vi "createPartsTracking.vi"(0 "reference in":refnum<class "PartsTracking Controller.lvclass">, 5 "error in (no error)":errorcluster) -> (14 "reference out":refnum<class "PartsTracking Controller.lvclass">, 19 "error out":errorcluster)   [LabVIEW 2016, in "PartsTracking Controller.lvclass"]
uses:
  PartsTracking Controller.lvclass
  APP/partsTracking_class/partsTracking.lvclass
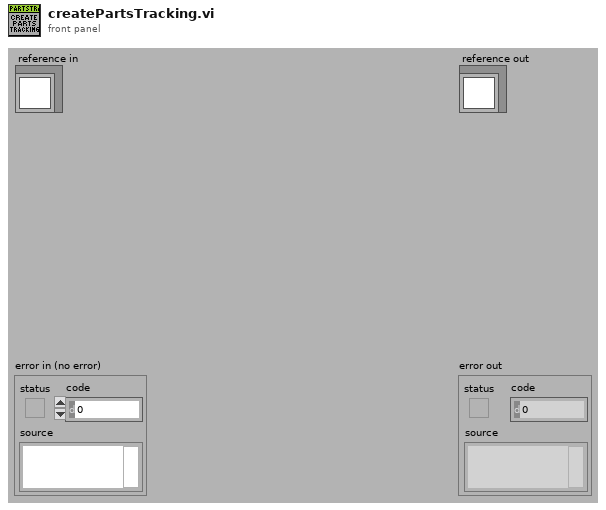
[diagram p1: front panel]
types:
  T1 = typedef "PartsTracking Controller.lvclass/ObjectAttributesRef.ctl" = refnum<data-value>
  T2 = typedef "PartsTracking Controller.lvclass/ObjectAttributes.ctl" = cluster{"MyAttribute":dbl, "file_controller_ref":refnum<class "File Controller.lvclass">, "data":string[][], "partsTracking_ref":refnum<class "partsTracking.lvclass">, "project_panels_ref":refnum<class "Project Panels.lvclass">}
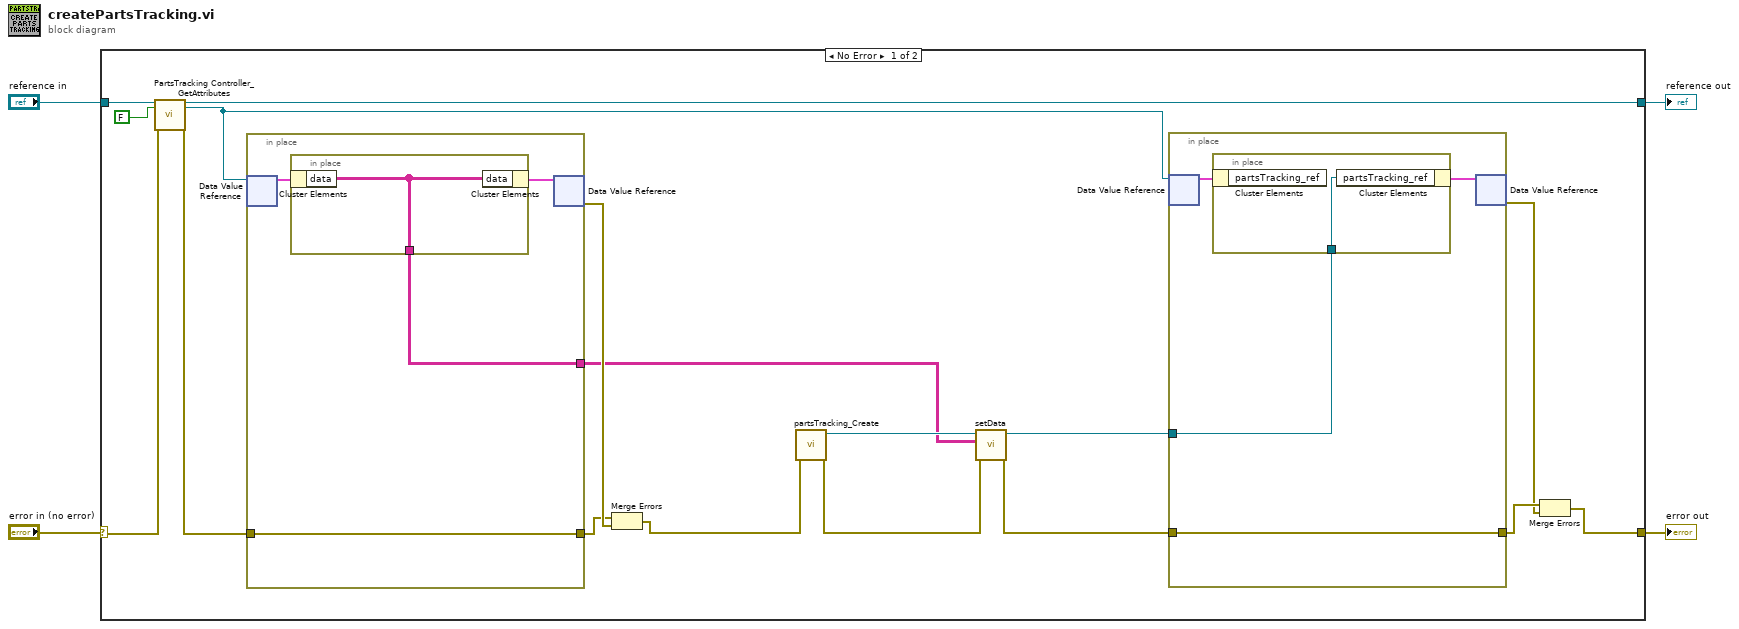
[diagram p0: block diagram]
diagram:
  n1 = case shown="No Error" "error in (no error)" {
    selector: "error in (no error)" -> [w17 w33]
    tunnel: [w11 w33] -> w3
    tunnel: [w15 w32] -> w1
    tunnel: "reference in" -> [w19 w32]
    frame No Error {
      n2 = call "PartsTracking Controller_GetAttributes.vi"("reference in"=w19, "return data? (T)"=FALSE, "error in (no error)"=w17) -> ("reference out"=w15:refnum<class "PartsTracking Controller.lvclass">, "attributes ref"=w10:T1, "error out"=w16:errorcluster)  [unwired: 13 in, 1 out]
      n3 = in-place {
        in-place-border: w16 -> [w28]
        in-place-border: [w28] -> w20
        in-place-border: [w27] -> w5
        n4 = in-place-dvr #1(w10) -> (w29:T2)  [unwired: 1 out]
        n5 = in-place {
          in-place-border: [w31] -> w27
          n6 = in-place-cluster #2(w29) -> ("data"=w31:string[][])
          n7 = in-place-cluster #2("data"=w31) -> (w30:T2)
        }
        n8 = in-place-dvr #1(w30) -> (w21:errorcluster)  [unwired: 1 out]
      }
      n9 = Merge Errors(w20, w21) -> (w14:errorcluster)
      n10 = call "partsTracking_Create.vi"("error in (no error)"=w14) -> ("error out"=w7:errorcluster, "reference out"=w9:refnum<class "partsTracking.lvclass">)  [unwired: 7 in]
      n11 = call "setData.vi"("error in (no error)"=w7, "data"=w5, "reference in"=w9) -> ("error out"=w6:errorcluster, "reference out"=w8:refnum<class "partsTracking.lvclass">)  [unwired: 7 in]
      n12 = in-place {
        in-place-border: w6 -> [w23]
        in-place-border: [w23] -> w13
        in-place-border: w8 -> [w22]
        n13 = in-place-dvr #3(w10) -> (w24:T2)  [unwired: 1 out]
        n14 = in-place {
          in-place-border: w22 -> [w26]
          n15 = in-place-cluster #4(w24) -> ()  [unwired: 1 out]
          n16 = in-place-cluster #4("partsTracking_ref"=w26) -> (w25:T2)
        }
        n17 = in-place-dvr #3(w25) -> (w12:errorcluster)  [unwired: 1 out]
      }
      n18 = Merge Errors(w13, w12) -> (w11:errorcluster)
    }
    frame Error {
    }
  }
  "error out" <- w3
  "reference out" <- w1
